vi "test Strip Class Function Name.vi"() -> ()   [LabVIEW 2017]
uses:
  String/Strip Class Function Name.vi/82d5ef48-2c95-4ac8-8452-541d4ca00c93.vi
  String/Strip Class Function Name.vi/8c0b350f-6b41-4dd8-8255-dad520baa4a5.vi
panel:
  out "library name 14":string
  out "Class name 14":string
  out "Function Name 14":string="replace memory subs"
  out "library name 13":string
  out "Class name 13":string
  out "Function Name 13":string="replace memory subs"
  out "library name 12":string
  out "Class name 12":string
  out "Function Name 12":string="replace memory subs"
  out "library name 11":string
  out "Class name 11":string
  out "Function Name 11":string="replace memory subs"
  out "library name 10":string
  out "Class name 10":string
  out "Function Name 10":string="replace memory subs"
  out "library name 9":string
  out "Class name 9":string
  out "Function Name 9":string="replace memory subs"
  out "library name 8":string
  out "Class name 8":string
  out "Function Name 8":string="replace memory subs"
  out "library name 7":string
  out "Class name 7":string
  out "Function Name 7":string="replace memory subs"
  out "library name 6":string
  out "Class name 6":string
  out "Function Name 6":string="replace memory subs"
  out "library name 5":string
  out "Class name 5":string
  out "Function Name 5":string="replace memory subs"
  out "library name 4":string
  out "Class name 4":string
  out "Function Name 4":string="replace memory subs"
  out "library name 3":string
  out "Class name 3":string
  out "Function Name 3":string="replace memory subs"
  out "library name 2":string
  out "Class name 2":string
  out "Function Name 2":string="replace memory subs"
  out "Function Name":string="replace memory subs"
  out "Class name":string
  out "library name":string
  # "classname.lvclass:funcname.vi"
  # "libpname.lvlibp"
  # "libpname.lvlibp:libname.lvlib:classname.lvclass:funcname.vi"
  # "libpname.lvlibp:funcname.vi"
  # "libpname.lvlibp:libname.lvlib"
  # "libname.lvlib:classname.lvclass:funcname.vi"
  # "libname.lvlib:classname.lvclass"
  # "libpname.lvlib:funcname.vi"
  # "libpname.lvlibp:classname.lvclass:funcname.vi"
  # "funcname.vi"
  # "libpname.lvlibp:libname.lvlib:classname.lvclass"
  # "classname.lvclass"
  # "libpname.lvlibp:classname.lvclass"
  # "libname.lvlib"
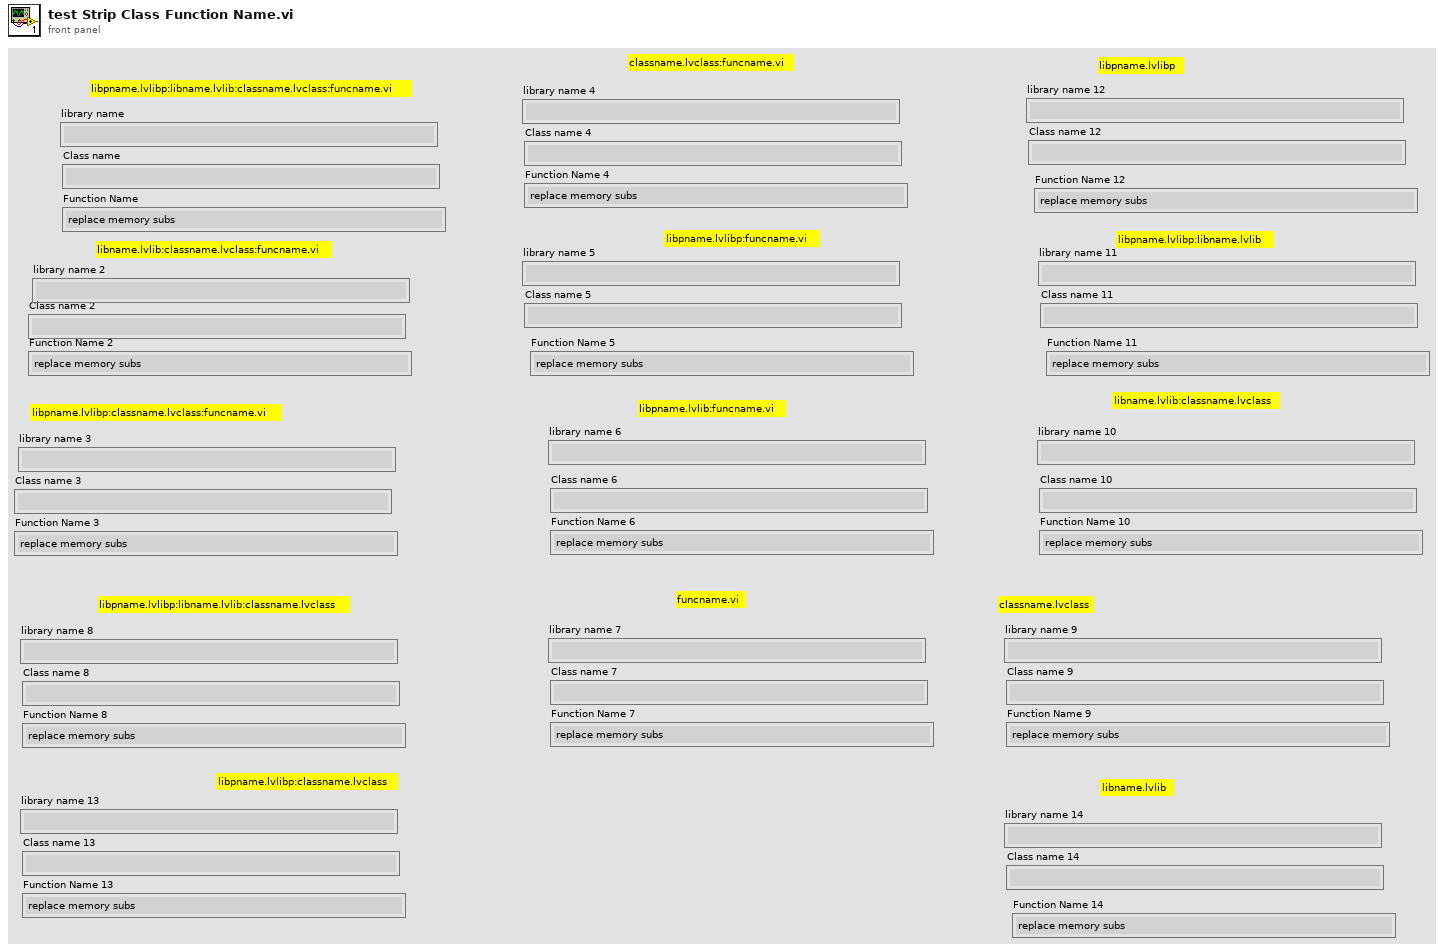
[diagram p1: front panel]
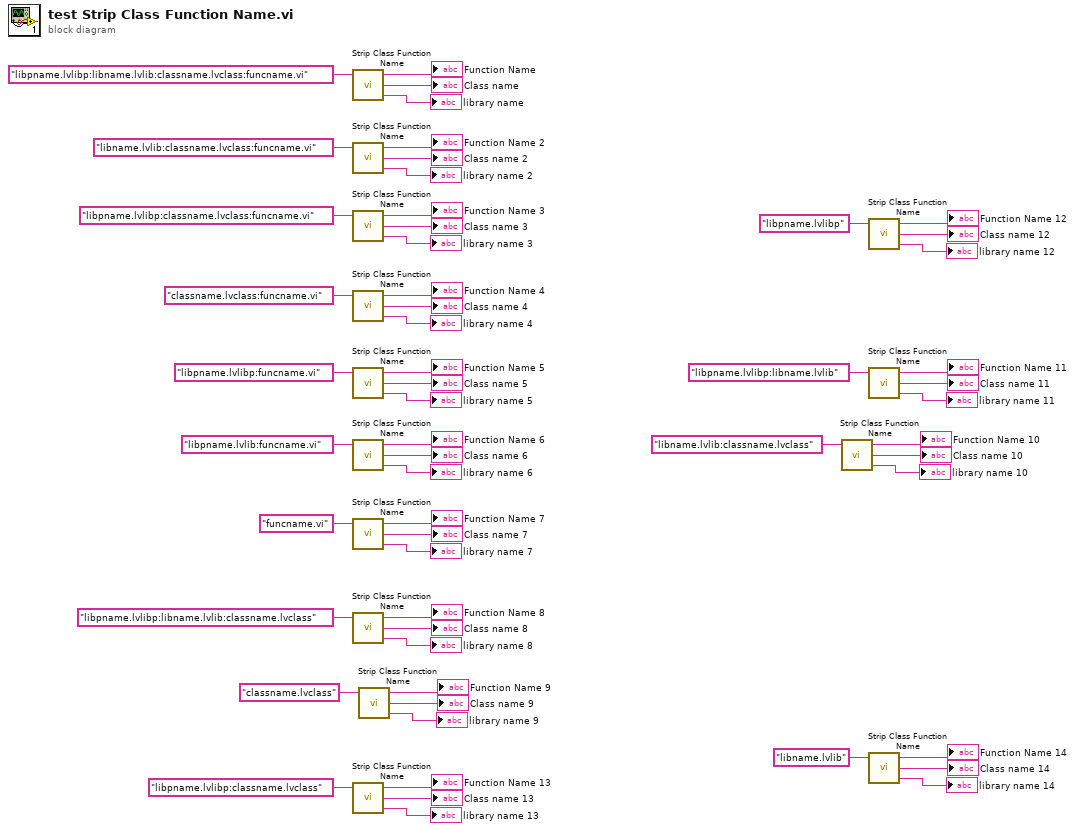
[diagram p0: block diagram]
diagram:
  n1 = call "Strip Class Function Name.vi"("File Full Path Name"="libpname.lvlibp:libname.lvlib:classname.lvclass:funcname.vi") -> ("library name"=→"library name":string, "Class name"=→"Class name":string, "Function Name"=→"Function Name":string)  [unwired: 2 in]
  n2 = call "Strip Class Function Name.vi"("File Full Path Name"="libname.lvlib:classname.lvclass:funcname.vi") -> ("library name"=→"library name 2":string, "Class name"=→"Class name 2":string, "Function Name"=→"Function Name 2":string)  [unwired: 2 in]
  n3 = call "Strip Class Function Name.vi"("File Full Path Name"="libpname.lvlibp:classname.lvclass:funcname.vi") -> ("library name"=→"library name 3":string, "Class name"=→"Class name 3":string, "Function Name"=→"Function Name 3":string)  [unwired: 2 in]
  n4 = call "Strip Class Function Name.vi"("File Full Path Name"="classname.lvclass:funcname.vi") -> ("library name"=→"library name 4":string, "Class name"=→"Class name 4":string, "Function Name"=→"Function Name 4":string)  [unwired: 2 in]
  n5 = call "Strip Class Function Name.vi"("File Full Path Name"="libpname.lvlibp:funcname.vi") -> ("library name"=→"library name 5":string, "Class name"=→"Class name 5":string, "Function Name"=→"Function Name 5":string)  [unwired: 2 in]
  n6 = call "Strip Class Function Name.vi"("File Full Path Name"="libpname.lvlib:funcname.vi") -> ("library name"=→"library name 6":string, "Class name"=→"Class name 6":string, "Function Name"=→"Function Name 6":string)  [unwired: 2 in]
  n7 = call "Strip Class Function Name.vi"("File Full Path Name"="funcname.vi") -> ("library name"=→"library name 7":string, "Class name"=→"Class name 7":string, "Function Name"=→"Function Name 7":string)  [unwired: 2 in]
  n8 = call "Strip Class Function Name.vi"("File Full Path Name"="libpname.lvlibp:libname.lvlib:classname.lvclass") -> ("library name"=→"library name 8":string, "Class name"=→"Class name 8":string, "Function Name"=→"Function Name 8":string)  [unwired: 2 in]
  n9 = call "Strip Class Function Name.vi"("File Full Path Name"="libpname.lvlibp:classname.lvclass") -> ("library name"=→"library name 13":string, "Class name"=→"Class name 13":string, "Function Name"=→"Function Name 13":string)  [unwired: 2 in]
  n10 = call "Strip Class Function Name.vi"("File Full Path Name"="classname.lvclass") -> ("library name"=→"library name 9":string, "Class name"=→"Class name 9":string, "Function Name"=→"Function Name 9":string)  [unwired: 2 in]
  n11 = call "Strip Class Function Name.vi"("File Full Path Name"="libname.lvlib:classname.lvclass") -> ("library name"=→"library name 10":string, "Class name"=→"Class name 10":string, "Function Name"=→"Function Name 10":string)  [unwired: 2 in]
  n12 = call "Strip Class Function Name.vi"("File Full Path Name"="libpname.lvlibp") -> ("library name"=→"library name 12":string, "Class name"=→"Class name 12":string, "Function Name"=→"Function Name 12":string)  [unwired: 2 in]
  n13 = call "Strip Class Function Name.vi"("File Full Path Name"="libpname.lvlibp:libname.lvlib") -> ("library name"=→"library name 11":string, "Class name"=→"Class name 11":string, "Function Name"=→"Function Name 11":string)  [unwired: 2 in]
  n14 = call "Strip Class Function Name.vi"("File Full Path Name"="libname.lvlib") -> ("library name"=→"library name 14":string, "Class name"=→"Class name 14":string, "Function Name"=→"Function Name 14":string)  [unwired: 2 in]
